vi "test-runge-kutta-time-varying.vi"(8 "error in (no error)":errorcluster) -> (0 "error out":errorcluster, 3 "Test Passed":bool)   [LabVIEW 2019]
uses:
  <vilib>/Analysis/Matrix/Datatypes/RealMatrix.ctl
  <vilib>/Rock Robotics/WPI/ThirdParty/JAS_Junk/TrajLib/Trajectory_Library.lvlib
  <vilib>/Analysis/Matrix/NI_Matrix.lvlib
panel:
  out "ApproxEquals":bool
  out "solution 5":T1
  out "XY Graph":cluster{dbl[], dbl[]}[](graph)
  out "Error":bool
  out "integrate 6":T1
  out "solution 6":T1
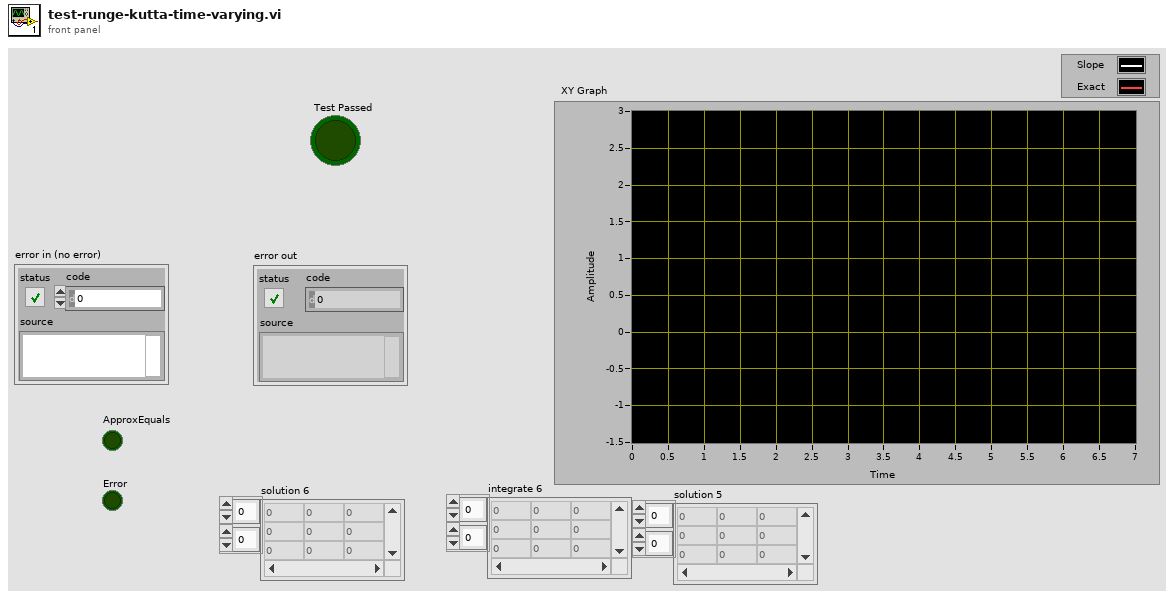
[diagram p1: front panel]
types:
  T1 = typedef "NI_Matrix.lvlib/RealMatrix.ctl" = dbl[][]
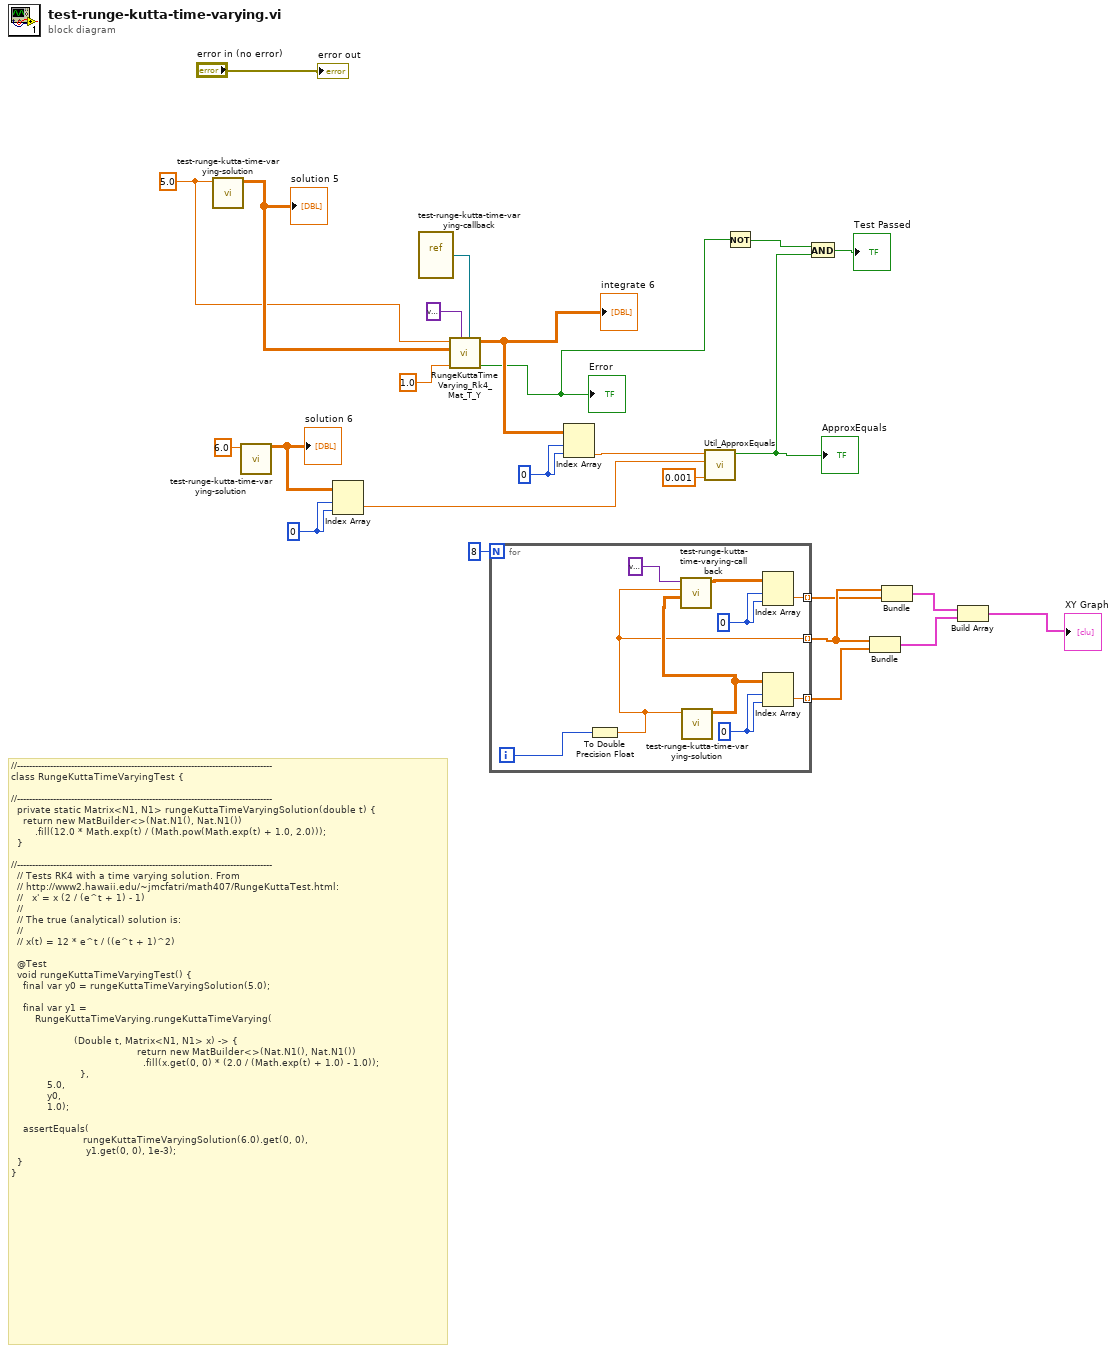
[diagram p0: block diagram]
diagram:
  w9 = 0 ("index (row)")
  w11 = 0 ("index (row)")
  w21 = 5.0 ("T")
  # "//-------------------------------------------------------------------------------------\nclass RungeKuttaTimeVaryingTest {\n\n//-------------------------------------------------------------------------------------\n  private static Matrix<N1, N1> rungeKuttaTimeVaryingSolution(double t) {\n    return new MatBuilder<>(Nat.N1(), Nat.N1())\n        .fill(12.0 * Math.exp(t) / (Math.pow(Math.exp(t) + 1.0, 2.0)));\n  }\n\n//-------------------------------------------------------------------------------------\n  // Tests RK4 with a time varying solution. From\n  // http://www2.hawaii.edu/~jmcfatri/math407/RungeKuttaTest.html:\n  //   x' = x (2 / (e^t + 1) - 1)\n  //\n  // The true (analytical) solution is:\n  //\n  // x(t) = 12 * e^t / ((e^t + 1)^2)\n\n  @Test\n  void rungeKuttaTimeVaryingTest() {\n    final var y0 = rungeKuttaTimeVaryingSolution(5.0);\n\n    final var y1 =\n        RungeKuttaTimeVarying.rungeKuttaTimeVarying(\n            \n                     (Double t, Matrix<N1, N1> x) -> {\n                                          return new MatBuilder<>(Nat.N1(), Nat.N1())\n                                            .fill(x.get(0, 0) * (2.0 / (Math.exp(t) + 1.0) - 1.0));\n                       },\n            5.0,\n            y0,\n            1.0);\n\n    assertEquals(\n                        rungeKuttaTimeVaryingSolution(6.0).get(0, 0), \n                         y1.get(0, 0), 1e-3);\n  }\n}"
  n1 = call "test-runge-kutta-time-varying-solution.vi"("T"=w21) -> ("output matrix"=w22:T1)  [unwired: 10 in]
  "solution 5" <- w22
  n2 = call "test-runge-kutta-time-varying-solution.vi"("T"=6.0) -> ("output matrix"=w10:T1)  [unwired: 10 in]
  "solution 6" <- w10
  n3 = Index Array(array=w10, index (row)=w11, index (col)=w11) -> (element=w6:dbl)
  n4 = vi-ref "test-runge-kutta-time-varying-callback.vi"() -> (w23:refnum<vi>)
  n5 = call <vilib>:"RungeKuttaTimeVarying_Rk4_Mat_T_Y.vi"("Func_T_Y_Extra"=w23, "PassedData"=variant, "dT_Seconds"=1.0, "Y"=w22, "T"=w21) -> ("Error"=w1:bool, "OUTPUT"=w8:T1)  [unwired: 5 in]
  "integrate 6" <- w8
  "Error" <- w1
  n6 = for {
    N: 8 -> [_]
    tunnel: [w29] -> w16 mode=indexing
    tunnel: [w32] -> w17 mode=indexing
    tunnel: [w26] -> w15 mode=indexing
    i -> [w34]
    w28 = 0 ("index (row)")
    w33 = 0 ("index (row)")
    n7 = To Double Precision Float(number=w34) -> (double precision float=w29:dbl)
    n8 = call "test-runge-kutta-time-varying-solution.vi"("T"=w29) -> ("output matrix"=w30:T1)  [unwired: 10 in]
    n9 = call "test-runge-kutta-time-varying-callback.vi"("Y"=w30, "T"=w29, "Variant"=variant) -> ("output matrix"=w27:T1)  [unwired: 7 in, 1 out]
    n10 = Index Array(array=w27, index (row)=w28, index (col)=w28) -> (element=w26:dbl)
    n11 = Index Array(array=w30, index (row)=w33, index (col)=w33) -> (element=w32:dbl)
  }
  n12 = Index Array(array=w8, index (row)=w9, index (col)=w9) -> (element=w7:dbl)
  n13 = call <vilib>:"Util_ApproxEquals.vi"("Tolerance"=0.001, "Value 2"=w6, "Value 1"=w7) -> ("ApproxEquals"=w3:bool)  [unwired: 8 in]
  "ApproxEquals" <- w3
  n14 = Not(x=w1) -> (.not. x?=w2:bool)
  n15 = And(x=w2, y=w3) -> (x .and. y?=→"Test Passed":bool)
  n16 = Bundle(w16, w17) -> (w13:cluster{dbl[], dbl[]})  [unwired: 1 in]
  n17 = Bundle(w16, w15) -> (w14:cluster{dbl[], dbl[]})  [unwired: 1 in]
  n18 = Build Array(w14, w13) -> (→"XY Graph":cluster{dbl[], dbl[]}[])
  "error out" <- "error in (no error)"
